vi "Right Level 2 Front Rocket.vi"() -> (4 "path":cluster{"X":dbl, "Y":dbl}[](array[cluster])=[{"X"=19.5, "Y"=112.0}, {"X"=20.500003415681597, "Y"=112.0000070643446}, {"X"=21.500015323999595, "Y"=112.00001435099331}, {"X"=22.500030428772963, "Y"=112.00001833581986}, {"X"=23.500041999365063, "Y"=112.00001676257503}, {"X"=24.500044765822935, "Y"=112.00000950248375}, {"X"=25.50003687006327, "Y"=111.9999984910794}, {"X"=26.5000202834009, "Y"=111.99998690451291}, {"X"=27.499999787752866, "Y"=111.99997799167765}, {"X"=28.499981116873776, "Y"=111.99997402363792}, {"X"=29.499969032604596, "Y"=111.99997569367008}, {"X"=30.499965984307515, "Y"=111.99998208745976}, {"X"=31.49997168305387, "Y"=111.99999113701797}, {"X"=32.49998356512972, "Y"=112.00000033907513}, {"X"=33.499997846737436, "Y"=112.00000748302107}, {"X"=34.50001074994158, "Y"=112.00001118183297}, {"X"=35.50001951183598, "Y"=112.00001109677403}, {"X"=36.50002292976273, "Y"=112.00000785283318}, {"X"=37.50002137860339, "Y"=112.0000027250824}, {"X"=38.500016398714735, "Y"=111.99999721937309}, {"X"=39.500010053048705, "Y"=111.99999267242123}, {"X"=40.5000042751706, "Y"=111.9999899659569}, {"X"=41.500000386895465, "Y"=111.99998940247691}, {"X"=42.49999888149069, "Y"=111.99999074166017}, {"X"=43.49999947699751, "Y"=111.99999335852299}, {"X"=44.50000137057765, "Y"=111.9999964633731}, {"X"=45.5000035846596, "Y"=111.99999932062008}, {"X"=46.50000529253045, "Y"=112.00000141536555}, {"X"=47.50000603805185, "Y"=112.00000253776567}, {"X"=48.50000580826017, "Y"=112.00000277905932}, {"X"=49.50000496408865, "Y"=112.00000245423453}, {"X"=50.50000407107624, "Y"=112.00000198060171}, {"X"=51.50000369138426, "Y"=112.00000174718961}, {"X"=52.50000419906065, "Y"=112.0000020071049}, {"X"=53.500005665487805, "Y"=112.0000028156446}, {"X"=54.500007837681714, "Y"=112.00000402392722}, {"X"=55.5000102059444, "Y"=112.00000532430909}, {"X"=56.5000121358139, "Y"=112.00000633273322}, {"X"=57.50001302659488, "Y"=112.0000066864238}, {"X"=58.500012456539935, "Y"=112.00000613387402}, {"X"=59.50001028192662, "Y"=112.00000459758888}, {"X"=60.50000667089035, "Y"=112.00000219730586}, {"X"=61.500002069042445, "Y"=111.99999923057133}, {"X"=62.4999971088017, "Y"=111.99999611656285}, {"X"=63.499992485034234, "Y"=111.9999933161425}, {"X"=64.49998882437777, "Y"=111.99999124506327}, {"X"=65.49998657433159, "Y"=111.99999019755401}, {"X"=66.49998593186885, "Y"=111.99999029443943}, {"X"=67.49998682187162, "Y"=111.99999146440386}, {"X"=68.49998892532867, "Y"=111.99999346025875}, {"X"=69.4999917480596, "Y"=111.99999590549186}, {"X"=70.49999471430071, "Y"=111.99999836118565}, {"X"=71.4999972666399, "Y"=112.00000040040429}, {"X"=72.49999895457834, "Y"=112.00000167671958}, {"X"=73.49999949781413, "Y"=112.00000197551257}, {"X"=74.49999881612139, "Y"=112.00000124047224}, {"X"=75.49999702417995, "Y"=111.99999957248461}, {"X"=76.49999439568398, "Y"=111.9999972029345}, {"X"=77.49999130558152, "Y"=111.99999444749363}, {"X"=78.49998816179682, "Y"=111.99999164912599}, {"X"=79.49998533811797, "Y"=111.99998912000082}, {"X"=80.4999831183356, "Y"=111.99998709127134}, {"X"=81.49998165869822, "Y"=111.9999856775513}, {"X"=82.49998097199273, "Y"=111.99998485989538}, {"X"=83.4999809327583, "Y"=111.99998448773567}, {"X"=84.49998129989078, "Y"=111.99998429712785}, {"X"=85.49998175063473, "Y"=111.99998394026575}, {"X"=86.49998191888288, "Y"=111.99998301981954}, {"X"=87.49998143080721, "Y"=111.99998112134816}, {"X"=88.49997993194003, "Y"=111.99997783772443}, {"X"=89.4999771015885, "Y"=111.99997278096114}, {"X"=90.49997265251824, "Y"=111.99996557870207}, {"X"=91.49996631583127, "Y"=111.99995585458018}, {"X"=92.49995781256052, "Y"=111.99994319331722}, {"X"=93.49994681451531, "Y"=111.99992709257721}, {"X"=94.49993289723011, "Y"=111.9999069040426}, {"X"=95.4999154875039, "Y"=111.99988176590914}, {"X"=96.49989380706492, "Y"=111.99985052802845}, {"X"=97.4998668125055, "Y"=111.99981166941764}, {"X"=98.4998331299784, "Y"=111.99976320593508}, {"X"=99.49979098138961, "Y"=111.99970258378082}, {"X"=100.4997380970856, "Y"=111.99962655223709}, {"X"=101.49967160838105, "Y"=111.99953100680834}, {"X"=102.49958791169577, "Y"=111.99941079164394}, {"X"=103.49948249463264, "Y"=111.99925944775825}, {"X"=104.49934971070785, "Y"=111.9990688911423}, {"X"=105.49918250515141, "Y"=111.99882899892394}, {"X"=106.49897197760738, "Y"=111.99852710371971}, {"X"=107.498707207683, "Y"=111.99814722663605}, {"X"=108.49837378431606, "Y"=111.99766964883439}, {"X"=109.49795507809971, "Y"=111.9970686233138}, {"X"=110.49742793374283, "Y"=111.9963137834679}, {"X"=111.49676545984704, "Y"=111.99536401906573}, {"X"=112.49593281760957, "Y"=111.99417032638603}, {"X"=113.49488566793725, "Y"=111.99267013989552}, {"X"=114.49356909875152, "Y"=111.99078379673873}, {"X"=115.49191413250664, "Y"=111.98841217712933}, {"X"=116.48983348303716, "Y"=111.98543098436768}, {"X"=117.48721735798019, "Y"=111.98168317890533}, {"X"=118.48392810258065, "Y"=111.9769710820088}, {"X"=119.47979278574282, "Y"=111.97104667826255}, {"X"=120.47459377618026, "Y"=111.96359845811018}, {"X"=121.46805728824567, "Y"=111.95423451511105}, {"X"=122.45983920000315, "Y"=111.94246180672755}, {"X"=123.44950706255685, "Y"=111.92766051848159}, {"X"=124.43651724626471, "Y"=111.90905168979113}, {"X"=125.42018617719978, "Y"=111.88565613108614}, {"X"=126.39965431828284, "Y"=111.8562426456282}, {"X"=127.37384100822331, "Y"=111.81926311973305}, {"X"=128.34138767328176, "Y"=111.77277114016661}, {"X"=129.3005863343288, "Y"=111.7143197097026}, {"X"=130.24928965101282, "Y"=111.64083251310281}, {"X"=131.18479783591658, "Y"=111.54844192897323}, {"X"=132.10371654346238, "Y"=111.4322853557438}, {"X"=133.00177825718572, "Y"=111.28624923660867}, {"X"=133.8736177360018, "Y"=111.10264733815534}, {"X"=134.7124896602979, "Y"=110.87181629801945}, {"X"=135.50991360454685, "Y"=110.58160708357286}, {"X"=136.25522766996346, "Y"=110.21674555750657}, {"X"=136.9640560624891, "Y"=109.7580285502104}, {"X"=137.64384595251443, "Y"=109.22465456540426}, {"X"=138.3005162074763, "Y"=108.63189303859795}, {"X"=138.9387687003952, "Y"=107.99188702641432}, {"X"=139.562336529715, "Y"=107.31429426554449}, {"X"=140.17417899983, "Y"=106.60679281914503}, {"X"=140.7766393315694, "Y"=105.87548771486753}, {"X"=141.371566491525, "Y"=105.12523106947123}, {"X"=141.96041261250218, "Y"=104.35987700306694}, {"X"=142.5443102213608, "Y"=103.58248527743606}, {"X"=143.12413148857772, "Y"=102.79548232432236}, {"X"=143.7005337037626, "Y"=102.00078849972795}, {"X"=144.27399413224757, "Y"=101.19991919230394}, {"X"=144.84483544601184, "Y"=100.3940648896611}, {"X"=145.4132425814961, "Y"=99.58415388604638}, {"X"=145.97927220831096, "Y"=98.77090094871484}, {"X"=146.54285569143718, "Y"=97.95484481983381}, {"X"=147.10379565831522, "Y"=97.13637663818614}, {"X"=147.66175572438598, "Y"=96.31576063698328}, {"X"=148.2162427297177, "Y"=95.4931480705189}, {"X"=148.7665806665707, "Y"=94.66858511447865}, {"X"=149.31187506792418, "Y"=93.842015249068}, {"X"=149.85096599875297, "Y"=93.01327630125745}, {"X"=150.38236708773078, "Y"=92.18209196130455}, {"X"=150.90418731152587, "Y"=91.34805726941744}, {"X"=151.41403141506143, "Y"=90.51061728396668}, {"X"=151.90887378497328, "Y"=89.66903783039133}, {"X"=152.38489919045082, "Y"=88.82236682995531}, {"X"=152.83730201465008, "Y"=87.96938419349269}, {"X"=153.2600333752557, "Y"=87.10853763402798}, {"X"=153.64548278595169, "Y"=86.23786099540732}, {"X"=153.98407759058753, "Y"=85.35487077938447}, {"X"=154.2692028616908, "Y"=84.4485627561135}, {"X"=154.5118021880318, "Y"=83.52371105785802}, {"X"=154.72058091373506, "Y"=82.58411381558629}, {"X"=154.90246432905778, "Y"=81.63279305783897}, {"X"=155.06296218235, "Y"=80.67215377290205}, {"X"=155.2064586818169, "Y"=79.70411049818102}, {"X"=155.3364432426426, "Y"=78.73018809197511}, {"X"=155.4556941271676, "Y"=77.75160199155805}, {"X"=155.56642465809725, "Y"=76.76932216039472}, {"X"=155.6703996746078, "Y"=75.78412424132365}, {"X"=155.76902856107773, "Y"=74.79662993903165}, {"X"=155.86343890944676, "Y"=73.80734109904644}, {"X"=155.95453738535352, "Y"=72.8166629923338}, {"X"=156.04305421859362, "Y"=71.82493101106427}, {"X"=156.12958672722928, "Y"=70.8324218536775}, {"X"=156.21462527121162, "Y"=69.83937284028985}, {"X"=156.29858225123576, "Y"=68.84599355108904}, {"X"=156.38181419488814, "Y"=67.85247498528054}, {"X"=156.4646385675773, "Y"=66.85900074575035}, {"X"=156.54735093516624, "Y"=65.8657575275312}, {"X"=156.6302416269073, "Y"=64.87294423431426}, {"X"=156.71361069400513, "Y"=63.88078189652282}, {"X"=156.79778296299304, "Y"=62.889525658375334}, {"X"=156.88312520459354, "Y"=61.89947866557172}, {"X"=156.97006595746953, "Y"=60.91100795052911}, {"X"=157.05911822092278, "Y"=59.924563401333266}, {"X"=157.15090614304532, "Y"=58.94070130432846}, {"X"=157.24619760419543, "Y"=57.96011378769359}, {"X"=157.3459447022246, "Y"=56.98366545230521}, {"X"=157.45133410772064, "Y"=56.01243889841933}, {"X"=157.56384964238728, "Y"=55.047791571909485}, {"X"=157.68535028388607, "Y"=54.091427089263796}, {"X"=157.81816784222883, "Y"=53.145484903543306}, {"X"=157.96522961862564, "Y"=52.2126530010664}, {"X"=158.1302125411588, "Y"=51.29630945882895}, {"X"=158.31773680082904, "Y"=50.40070024469594}, {"X"=158.53360907325504, "Y"=49.53116262899132}, {"X"=158.78512809529175, "Y"=48.69440602632272}, {"X"=159.08146872795567, "Y"=47.89886510029208}, {"X"=159.4341647907107, "Y"=47.155143722838375}, {"X"=159.85771611464145, "Y"=46.47657312346403}, {"X"=160.37361595678075, "Y"=45.83775607139759}, {"X"=160.9629688707403, "Y"=45.23055911221765}, {"X"=161.6107454244133, "Y"=44.648513020407044}, {"X"=162.3049911519145, "Y"=44.086472281119754}, {"X"=163.03619732666849, "Y"=43.540344258925415}, {"X"=163.79680046903235, "Y"=43.00687380485811}, {"X"=164.58078426461086, "Y"=42.48347195565298}, {"X"=165.38336293789794, "Y"=41.96807969388639}, {"X"=166.20072940641728, "Y"=41.459059582283174}, {"X"=167.02985489562124, "Y"=40.95510959546084}, {"X"=167.86832966679663, "Y"=40.455194482610246}, {"X"=168.71423575286374, "Y"=39.958491571069615}, {"X"=169.56604694818924, "Y"=39.46434668978945}, {"X"=170.42254687118592, "Y"=38.9722412246221}, {"X"=171.28276674990747, "Y"=38.48176274173707}, {"X"=172.14593334913823, "Y"=37.9925853111439}, {"X"=173.0114281071923, "Y"=37.504451356145886}, {"X"=173.878755393109, "Y"=37.01715781464259}, {"X"=174.7475162398843, "Y"=36.53054616534282}, {"X"=175.6173868062861, "Y"=36.04449392411508}, {"X"=176.4881015228044, "Y"=35.55890781442052}, {"X"=177.35943950051208, "Y"=35.0737190055596}, {"X"=178.2312127904785, "Y"=34.58887971565129}, {"X"=179.1032561722028, "Y"=34.10436062267383}, {"X"=179.97541845507078, "Y"=33.620149176452934}, {"X"=180.8475547712534, "Y"=33.13624896084246}, {"X"=181.71951907206866, "Y"=32.65267998597327}, {"X"=182.5911563151778, "Y"=32.16947976136023}, {"X"=183.462294140189, "Y"=31.68670520471644}, {"X"=184.33273378997424, "Y"=31.20443558953104}, {"X"=185.2022397687844, "Y"=30.72277673491863}, {"X"=186.0705275346787, "Y"=30.24186661745866}, {"X"=186.93724849346145, "Y"=29.76188264683413}, {"X"=187.80197155795634, "Y"=29.283050983386442}, {"X"=188.66416040581356, "Y"=28.805658420306948}, {"X"=189.5231452826728, "Y"=28.330067479862244}, {"X"=190.37808782547802, "Y"=27.85673551188412}, {"X"=191.22793698459373, "Y"=27.386238777653777}, {"X"=192.07137369154825, "Y"=26.919302774282514}, {"X"=192.90674138183843, "Y"=26.456840402180326}, {"X"=193.7319587628866, "Y"=26.0}], 6 "Reverse Path?":bool)   [LabVIEW 2018]
uses:
  AutonBuilder/Typedef/Data Point.ctl
panel:
  in  "Data Points":T1[](array[typedef])=[{"X"=19.5, "Y"=112.0, "Theta"=0.0, "Speed %"=0.0, "Disabled?"=FALSE}, {"X"=136.94845360824743, "Y"=112.0, "Theta"=0.0, "Speed %"=0.0, "Disabled?"=FALSE}, {"X"=155.0, "Y"=85.79790940766551, "Theta"=0.0, "Speed %"=0.0, "Disabled?"=FALSE}, {"X"=158.10309278350516, "Y"=45.721254355400696, "Theta"=0.0, "Speed %"=0.0, "Disabled?"=FALSE}, {"X"=193.7319587628866, "Y"=26.0, "Theta"=0.0, "Speed %"=0.0, "Disabled?"=FALSE}]
  out "Graph":cluster{dbl[], dbl[]}[](graph)=[{[0.0, 33.5, 33.5, 0.0, 0.0], [126.25, 126.25, 97.75, 97.75, 126.25]}, {[19.5, 136.94845360824743, 155.0, 158.10309278350516, 193.7319587628866], [112.0, 112.0, 85.79790940766551, 45.721254355400696, 26.0]}, {array[233 elements], array[233 elements]}, {array[233 elements], array[233 elements]}, {array[233 elements], array[233 elements]}]
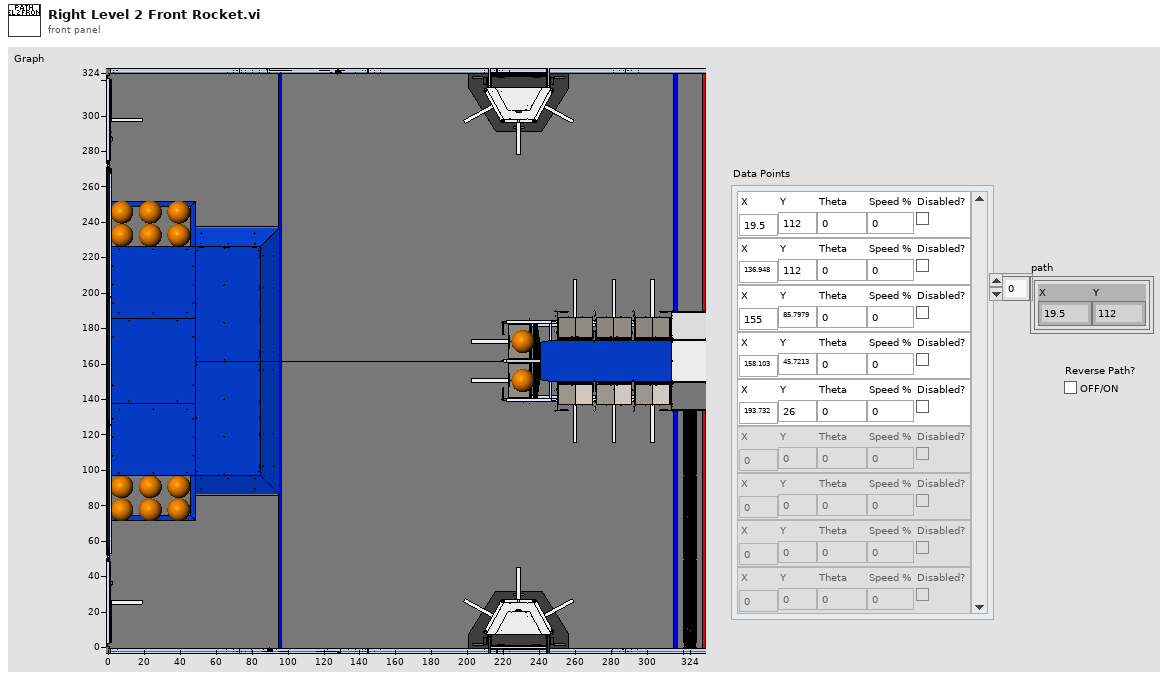
[diagram p1: front panel]
types:
  T1 = typedef "Data Point.ctl" = cluster{"X":dbl, "Y":dbl, "Theta":dbl, "Speed %":dbl, "Disabled?":bool}
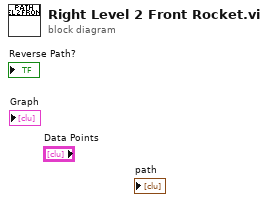
[diagram p0: block diagram]
diagram:
